vi "Spatial Dual Main (VISA).vi"(6 "Queue in":refnum<queue>, 7 "error in":errorcluster) -> (0 "error out":errorcluster)   [LabVIEW 2019]
uses:
  Globals and Definitions/System Message.ctl
  Globals and Definitions/Serial - Settings.ctl
  Globals and Definitions/Enum_FileNewInterval.ctl
  Globals and Definitions/RT Globals RD v1.0.vi
  <vilib>/Instr/_visa.llb/VISA Configure Serial Port (Instr).vi
  Globals and Definitions/Initialization Globals.vi
  <vilib>/Utility/file.llb/Write Delimited Spreadsheet (string).vi
  SpatialDual_Parsers.lvlib
panel:
  in  "Read Count":u32=1000
  in  "Termination Character":u8=10 format="%.0x"
  in  "VISA resource name":refnum<visa-resource-name>="COM1"
  in  "Serial Settings":T1={"baud rate"=9600, "data bits"=8, "parity"=enum."None", "stop bits"=10, "flow control"=0} {"flow control" items=["None"=0, "XON/XOFF"=1, "RTS/CTS"=2, "DTR/DSR"=4]; "stop bits" items=["1.0"=10, "1.5"=15, "2.0"=20]; "data bits" min=5 max=8 step=1; "baud rate" items=["75"=75, "110"=110, "134"=134, "150"=150, "300"=300, "600"=600, "1200"=1200, "1800"=1800, "2400"=2400, "4800"=4800, "7200"=7200, "9600"=9600, "14400"=14400, "19200"=19200, "28800"=28800, "38400"=38400, "56000"=56000, "57600"=57600, "115200"=115200, "128000"=128000, "230400"=230400]}
  out "Unix Timestamp":u64
  out "INS Filter Status Array":bool[](array[boolean])
  out "Packet 20 Decoded Data Cluster":T2
  in  "String Precision":i16=6
  out "size(s)":i32
  out "Packet Size":u8
  out "Packet ID":u8
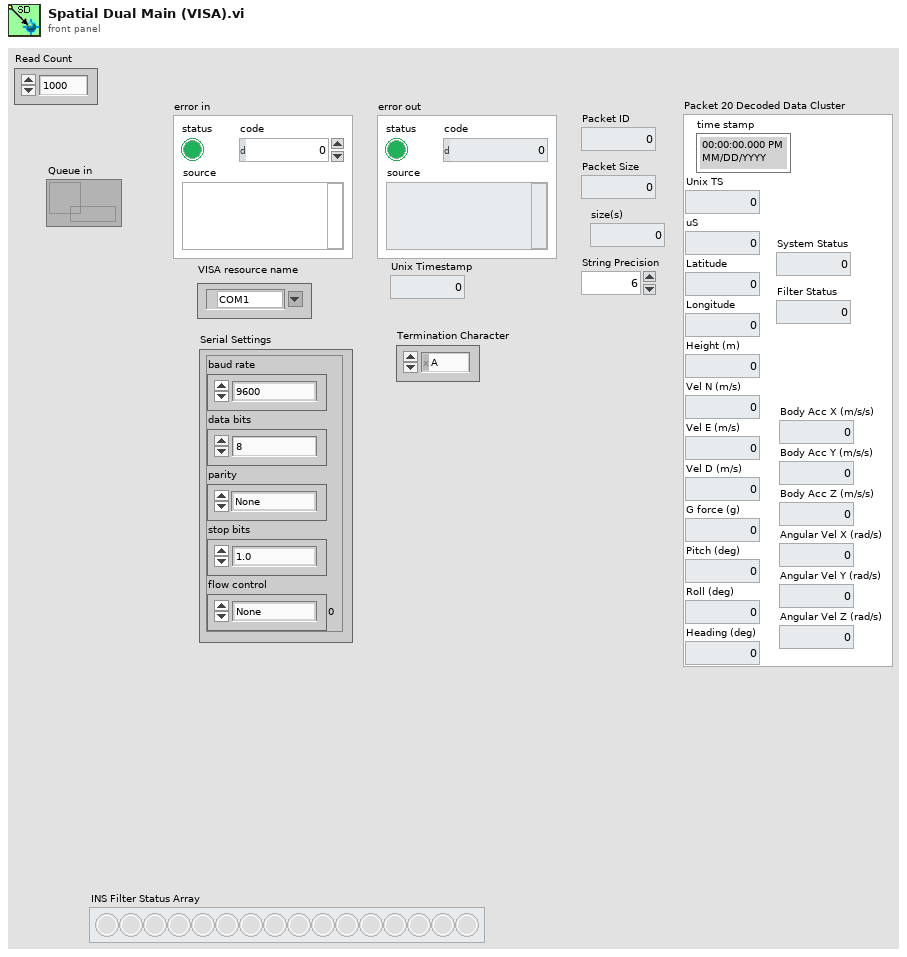
[diagram p1: front panel]
types:
  T1 = typedef "Serial - Settings.ctl" = cluster{"baud rate":u32, "data bits":u16, "parity":enum16{"None", "Odd", "Even", "Mark", "Space"}, "stop bits":u16, "flow control":u16}
  T2 = cluster{"time stamp":timestamp, "Unix TS":u32, "uS":u32, "Latitude":dbl, "Longitude":dbl, "Height (m)":dbl, "Vel N (m/s)":sgl, "Vel E (m/s)":sgl, "Vel D (m/s)":sgl, "G force (g)":sgl, "Pitch (deg)":sgl, "Roll (deg)":sgl, "Heading (deg)":sgl, "Body Acc X (m/s/s)":sgl, "Body Acc Y (m/s/s)":sgl, "Body Acc Z (m/s/s)":sgl, "Angular Vel X (rad/s)":sgl, "Angular Vel Y (rad/s)":sgl, "Angular Vel Z (rad/s)":sgl, "Filter Status":u16, "System Status":u16}
  T3 = enum16{"CRC Check", "Load Packet", "LRC Check", "Prescan Stream"}
  T4 = typedef "System Message.ctl" = cluster{"Message Tag":string, "Message Body":string, "Snooze Time (s)":dbl, "Snooze Alert?":bool, "Log Event?":bool, "Send Email":i32}
  T5 = typedef "Enum_FileNewInterval.ctl" = enum16{"10 Min", "Hourly", "Daily", "Weekly", "Monthly"}
  T6 = cluster{"All Data Types":string[], "All Units":string[], "All Names":string[], "Group Name":string}
  T7 = cluster{"Unix TS":u32, "uS":u32, "Latitude":dbl, "Longitude":dbl, "Height (m)":dbl, "Vel N (m/s)":sgl, "Vel E (m/s)":sgl, "Vel D (m/s)":sgl, "G force (g)":sgl, "Pitch (deg)":sgl, "Roll (deg)":sgl, "Heading (deg)":sgl, "Body Acc X (m/s/s)":sgl, "Body Acc Y (m/s/s)":sgl, "Body Acc Z (m/s/s)":sgl, "Angular Vel X (rad/s)":sgl, "Angular Vel Y (rad/s)":sgl, "Angular Vel Z (rad/s)":sgl, "Filter Status":u16, "System Status":u16}
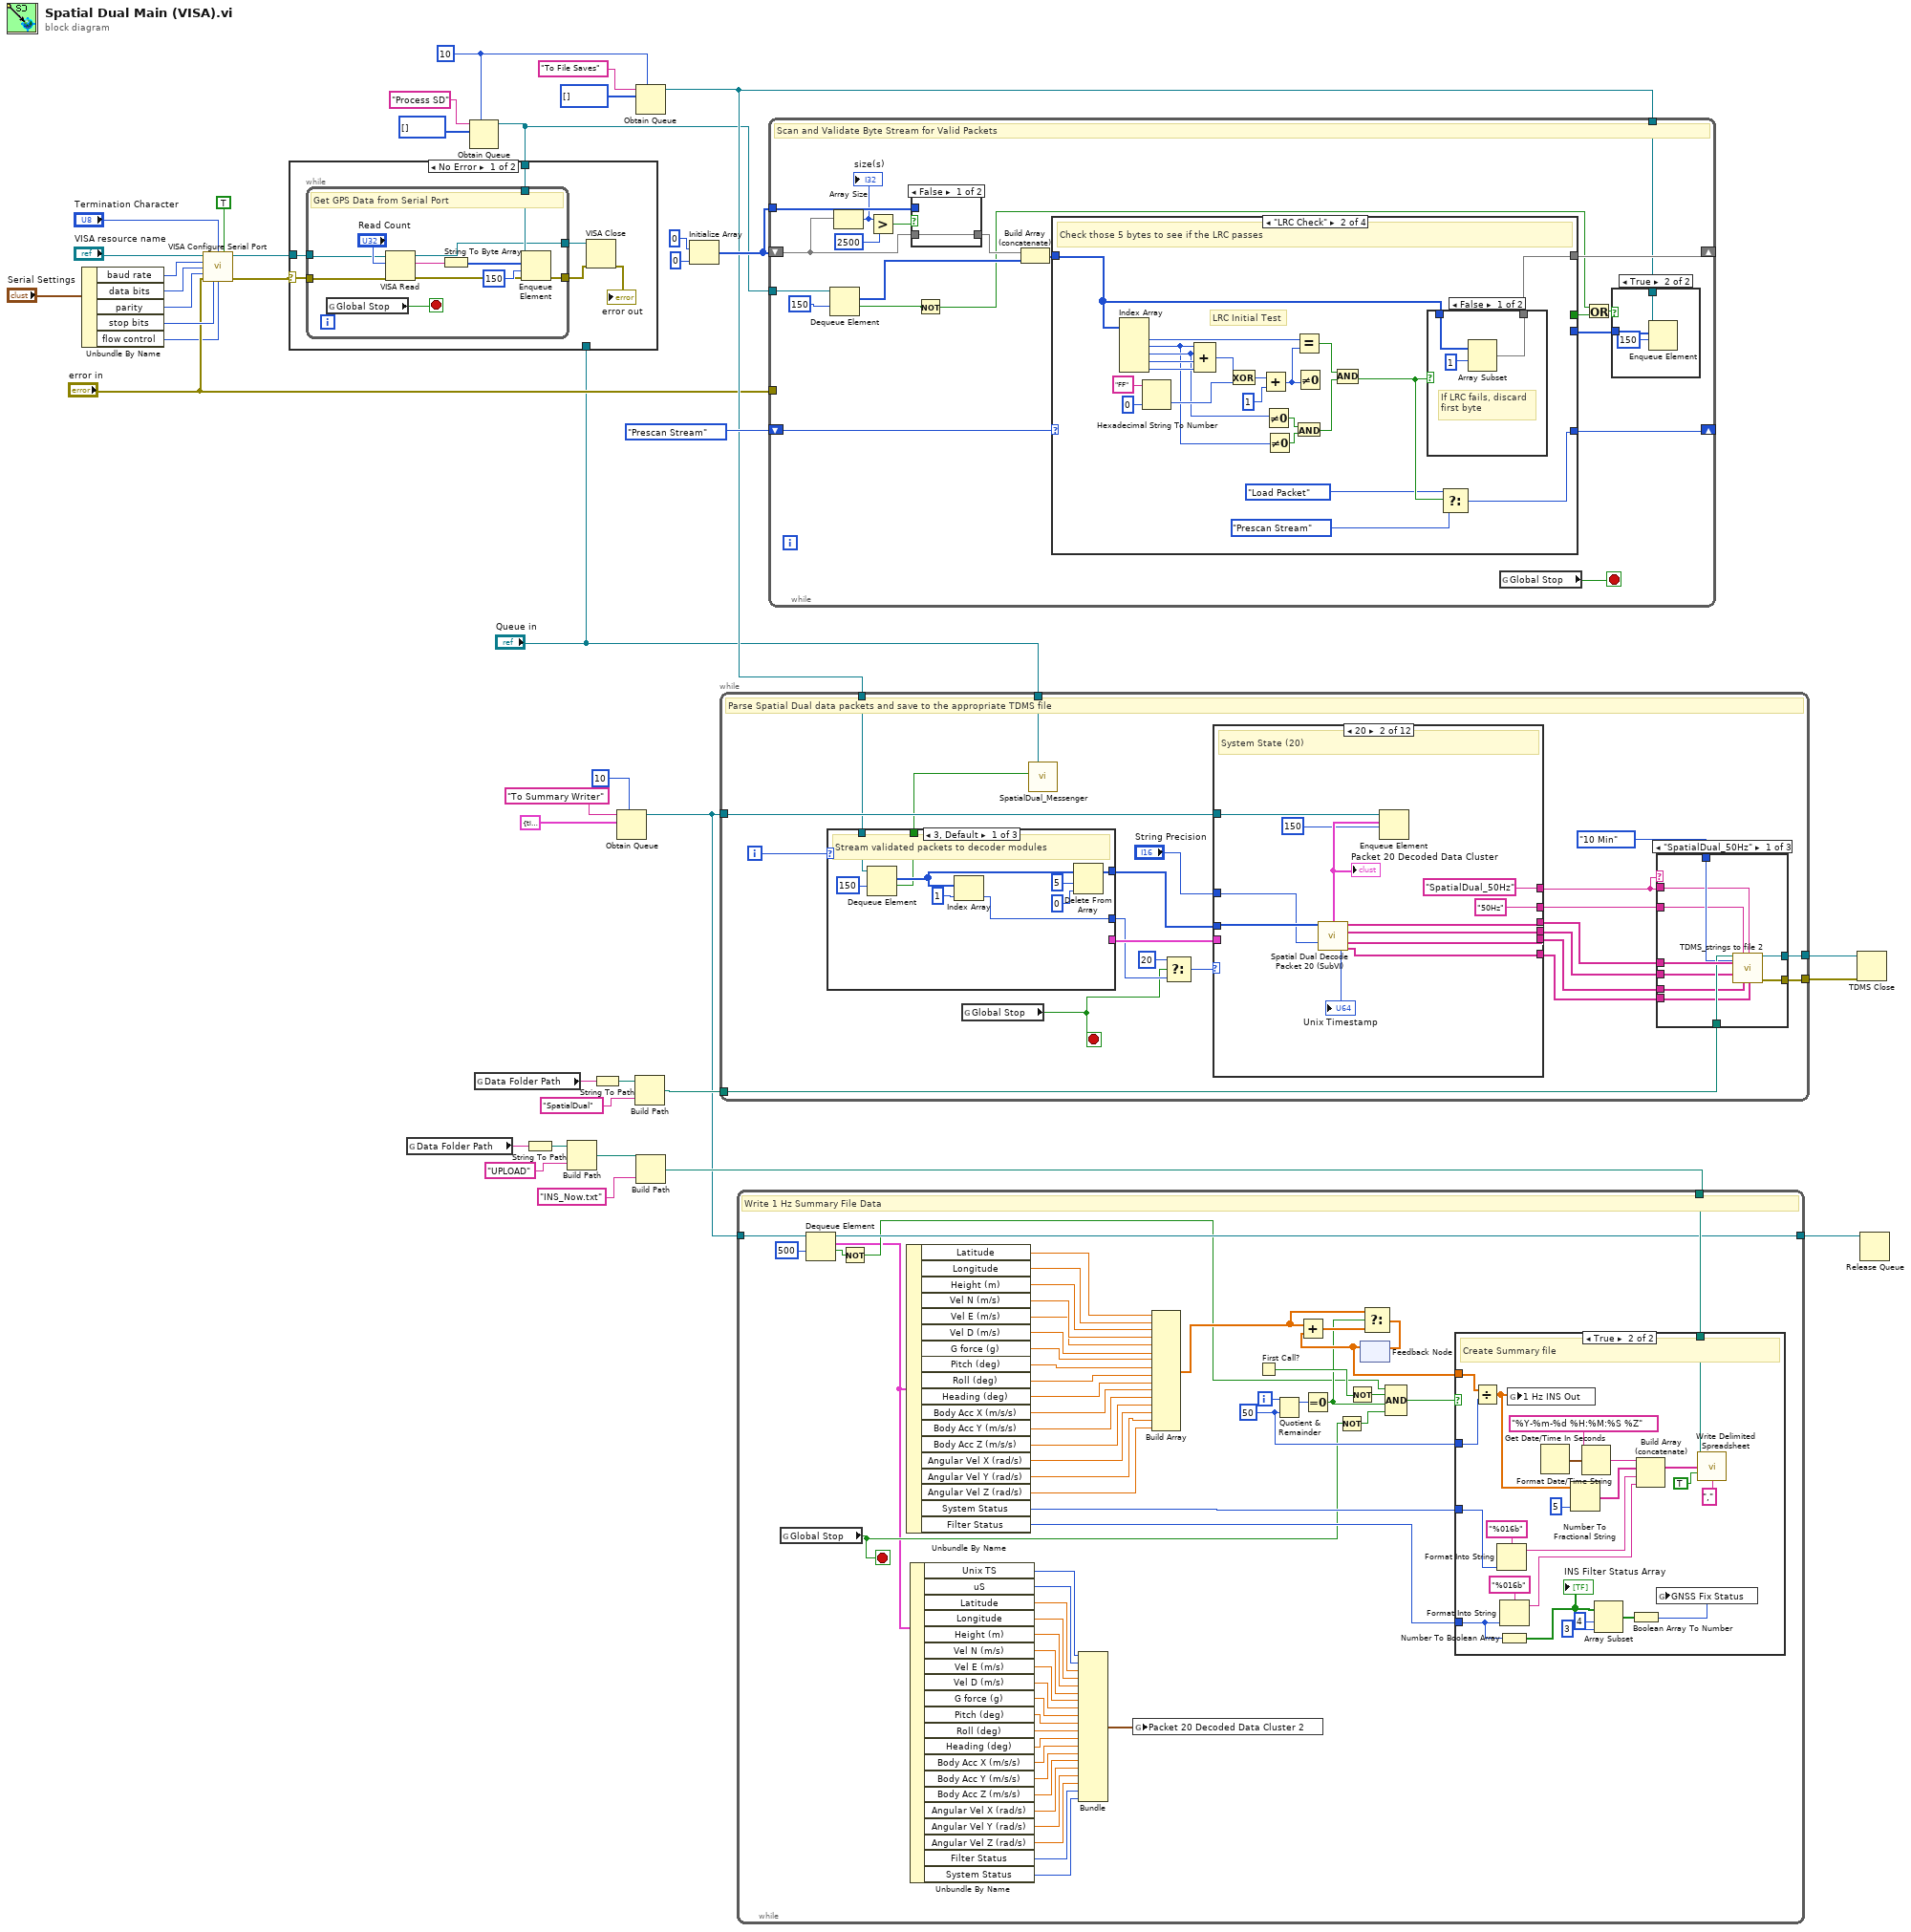
[diagram p0: block diagram]
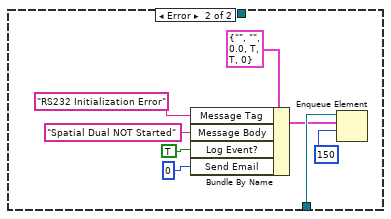
[diagram p2: hidden frame]
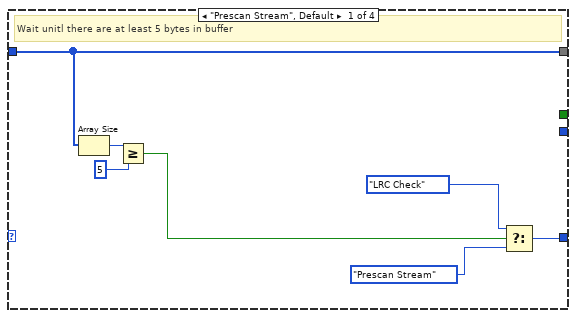
[diagram p6: hidden frame]
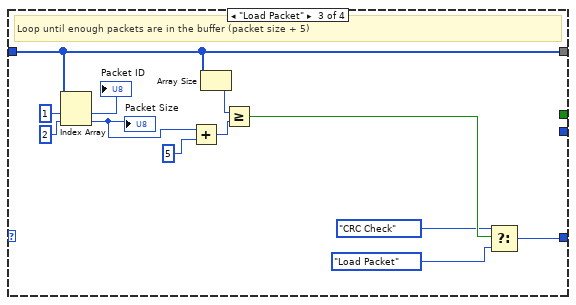
[diagram p8: hidden frame]
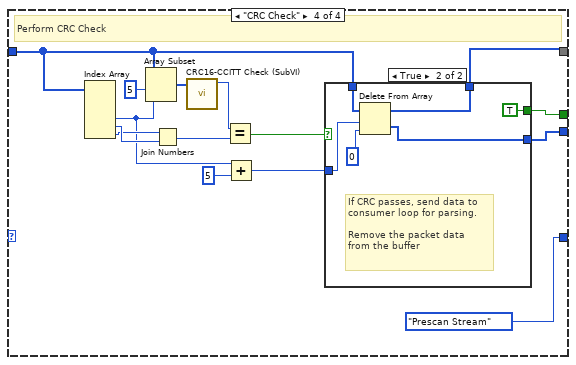
[diagram p9: hidden frame]
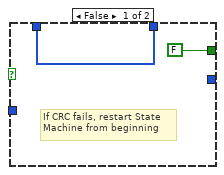
[diagram p10: hidden frame]
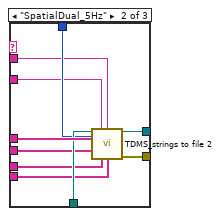
[diagram p11: hidden frame]
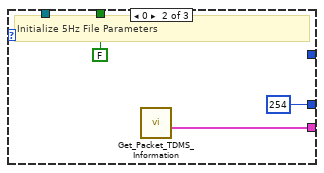
[diagram p13: hidden frame]
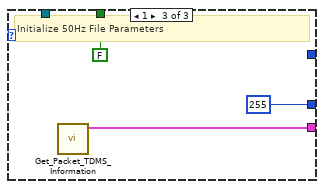
[diagram p14: hidden frame]
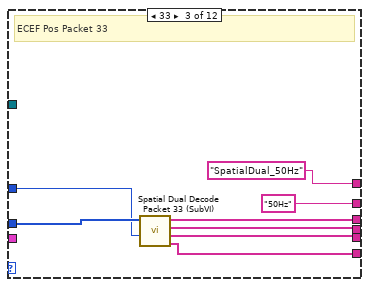
[diagram p16: hidden frame]
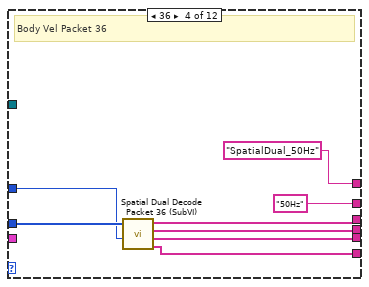
[diagram p17: hidden frame]
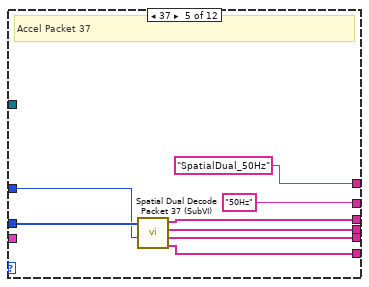
[diagram p18: hidden frame]
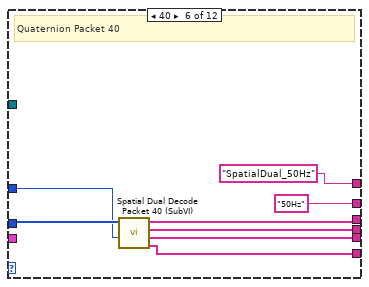
[diagram p19: hidden frame]
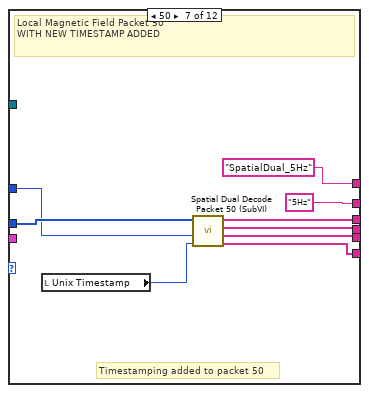
[diagram p20: hidden frame]
diagram:
  w15 = 10 ("max queue size (-1, unlimited)")
  n1 = Unbundle By Name("Serial Settings") -> ("baud rate"=w12:u32, "data bits"=w11:u16, "parity"=w10:enum16{"None", "Odd", "Even", "Mark", "Space"}, "stop bits"=w9:u16, "flow control"=w4:u16)
  n2 = call-poly "VISA Configure Serial Port"("VISA resource name"="VISA resource name", "termination char\n(0xA = '\\n' = LF)"="Termination Character", "Enable Termination\nChar (T)"=TRUE ("Enable Termination\nChar (T)"), "baud rate (9600)"=w12, "data bits (8)"=w11, "parity (0:none)"=w10, "error in (no error)"="error in", "stop bits (10: 1 bit)"=w9, "flow control (0:none)"=w4) -> ("VISA resource name out"=w3:refnum<visa-resource-name>, "error out"=w2:errorcluster)  [unwired: 1 in, 4 out]
  n3 = global read "Initialization Globals.vi" "Data Folder Path"() -> (w29:string)
  n4 = Obtain Queue(max queue size (-1, unlimited)=w15, name (unnamed)="Process SD", element data type=u8[] [] ("appended array")) -> (queue out=w16:refnum<queue>)  [unwired: 2 in, 2 out]
  n5 = case shown="No Error" w2 {
    selector: w2 -> [w42 _]
    tunnel: w16 -> [w47 _]
    tunnel: w3 -> [w46 _]
    tunnel: "Queue in" -> [_ w63]
    frame No Error {
      n6 = while {
        tunnel: w47 -> [w57]
        tunnel: w42 -> [w51]
        tunnel: w46 -> [w54]
        tunnel: [w49] -> w45
        tunnel: [w48] -> w44
        stop <- w58 stop-if-true
        # "Get GPS Data from Serial Port"
        n7 = global read "RT Globals RD v1.0.vi" "Global Stop"() -> (w58:bool)
        n8 = VISA Read(VISA resource name=w54, byte count="Read Count", error in (no error)=w51) -> (VISA resource name out=w49:refnum<visa-resource-name>, read buffer=w53:string, error out=w50:errorcluster)  [unwired: 1 out]
        n9 = String To Byte Array(string=w53) -> (unsigned byte array=w52:u8[])
        n10 = Enqueue Element(queue=w57, element=w52, timeout in ms (-1)=150, error in (no error)=w50) -> (error out=w48:errorcluster)  [unwired: 2 out]
      }
      n11 = VISA Close(VISA resource name=w45, error in (no error)=w44) -> (error out=→"error out":errorcluster)
    }
    frame Error {
      n12 = Bundle By Name(cluster=T4 {"Message Tag"="", "Message Body"="", "Snooze Time (s)"=0.0, "Snooze Alert?"=TRUE, "Log Event?"=TRUE, "Send Email"=0}, "Message Tag"="RS232 Initialization Error", "Message Body"="Spatial Dual NOT Started", "Log Event?"=TRUE, "Send Email"=0) -> (w62:T4)
      n13 = Enqueue Element(queue=w63, element=w62, timeout in ms (-1)=150) -> ()  [unwired: 1 in, 3 out]
    }
  }
  n14 = global read "Initialization Globals.vi" "Data Folder Path"() -> (w33:string)
  n15 = String To Path(string=w29) -> (path=w30:path)
  n16 = Build Path(base path=w30, name or relative path="UPLOAD") -> (appended path=w27:path)
  n17 = String To Path(string=w33) -> (path=w34:path)
  n18 = Obtain Queue(max queue size (-1, unlimited)=10, name (unnamed)="To Summary Writer", element data type=T2 {"time stamp"=timestamp(0 s since 1904-01-01), "Unix TS"=0, "uS"=0, "Latitude"=0.0, "Longitude"=0.0, "Height (m)"=0.0, "Vel N (m/s)"=0.0, "Vel E (m/s)"=0.0, "Vel D (m/s)"=0.0, "G force (g)"=0.0, "Pitch (deg)"=0.0, "Roll (deg)"=0.0, "Heading (deg)"=0.0, "Body Acc X (m/s/s)"=0.0, "Body Acc Y (m/s/s)"=0.0, "Body Acc Z (m/s/s)"=0.0, "Angular Vel X (rad/s)"=0.0, "Angular Vel Y (rad/s)"=0.0, "Angular Vel Z (rad/s)"=0.0, "Filter Status"=0, "System Status"=0} ("Packet 20 Decoded Data Cluster 2")) -> (queue out=w24:refnum<queue>)  [unwired: 2 in, 2 out]
  n19 = Build Path(base path=w34, name or relative path="SpatialDual") -> (appended path=w32:path)
  n20 = Obtain Queue(max queue size (-1, unlimited)=w15, name (unnamed)="To File Saves", element data type=u8[] []) -> (queue out=w19:refnum<queue>)  [unwired: 2 in, 2 out]
  n21 = Build Path(base path=w27, name or relative path="INS_Now.txt") -> (appended path=w26:path)
  n22 = Initialize Array(u8 0, 0 ("dimension size")) -> (w39:u8[])
  n23 = while {
    tunnel: w32 -> [w84]
    tunnel: [w87] -> w37
    tunnel: [w86] -> w36
    tunnel: w24 -> [w71]
    tunnel: "Queue in" -> [w69]
    tunnel: w19 -> [w68]
    i -> [w76]
    stop <- w67 stop-if-true
    # "Parse Spatial Dual data packets and save to the appropriate TDMS file"
    n24 = case shown="3, Default" w76 {
      tunnel: [w114 _ _] -> w88
      tunnel: [w113 u8 254 u8 255] -> w72
      tunnel: [_ w120 w122] -> w77
      tunnel: [w110 FALSE ("timed out?") FALSE ("timed out?")] -> w70
      tunnel: w68 -> [w112 _ _]
      frame 3, Default {
        # "Stream validated packets to decoder modules"
        n25 = Dequeue Element(queue=w112, timeout in ms (-1)=150) -> (element=w111:u8[], timed out?=w110:bool)  [unwired: 1 in, 2 out]
        n26 = Index Array(array=w111, index=1) -> (element=w113:u8)
        n27 = Delete From Array(array=w111, length=5, index=0) -> (array with subset deleted=w114:u8[])  [unwired: 1 out]
      }
      frame 0 {
        # "Initialize 5Hz File Parameters"
        n28 = call "Get_Packet_TDMS_Information.vi"() -> ("TDMS Info 5Hz"=w120:T6)  [unwired: 10 in, 1 out]
      }
      frame 1 {
        # "Initialize 50Hz File Parameters"
        n29 = call "Get_Packet_TDMS_Information.vi"() -> ("TDMS Info 50Hz"=w122:T6)  [unwired: 10 in, 1 out]
      }
    }
    n30 = global read "RT Globals RD v1.0.vi" "Global Stop"() -> (w67:bool)
    n31 = call "SpatialDual_Messenger.vi"("Queue in"=w69, "Time Out"=w70) -> ()  [unwired: 10 in]
    n32 = Select(t=20, s=w67, f=w72) -> (s? t:f=w74:i32)
    n33 = case shown="20" w74 {
      tunnel: w88 -> [_ w135 w143 w151 w159 w167 w175 w183 w191 w200 _ _]
      tunnel: [_ w134 w141 w149 w158 w165 w173 w181 w189 w198 w204 w212] -> w85
      tunnel: [_ w133 w140 w148 w157 w164 w172 w180 w188 w197 _ _] -> w83
      tunnel: [_ w132 w139 w147 w156 w163 w171 w179 w187 w196 w203 w211] -> w82
      tunnel: [_ w131 w138 w146 w155 w162 w170 w178 w186 w195 w202 w210] -> w81
      tunnel: [_ "50Hz" ("FileName") "50Hz" ("FileName") "50Hz" ("FileName") "50Hz" ("FileName") "50Hz" ("FileName") "5Hz" ("FileName") "5Hz" ("FileName") "50Hz" ("FileName") "5Hz" ("FileName") w205 w209] -> w79
      tunnel: "String Precision" -> [_ w129 w142 w150 w153 w166 w174 w182 w190 w199 _ _]
      tunnel: w77 -> [_ _ _ _ _ _ _ _ _ _ w206 w207]
      tunnel: [_ "SpatialDual_50Hz" ("FileName") "SpatialDual_50Hz" ("FileName") "SpatialDual_50Hz" ("FileName") "SpatialDual_50Hz" ("FileName") "SpatialDual_50Hz" ("FileName") "SpatialDual_5Hz" ("FileName") "SpatialDual_5Hz" ("FileName") "SpatialDual_50Hz" ("FileName") "SpatialDual_5Hz" ("FileName") "SpatialDual_5Hz" ("FileName") "SpatialDual_50Hz" ("FileName")] -> w75
      tunnel: w71 -> [_ w127 _ _ _ _ _ _ _ _ _ _]
      frame 0, Default {
      }
      frame 20 {
        # "System State (20)"
        n34 = call "Spatial Dual Decode Packet 20 (SubVI).vi"("Packet 20 Bytes In"=w135, "String Precision"=w129) -> ("Packet 20 Decoded Data Cluster"=w126:T2, "Channel Names"=w134:string[], "Data"=w133:string[], "Channel Units"=w132:string[], "Unix Timestamp"=→"Unix Timestamp":u64, "Data Types"=w131:string[])  [unwired: 8 in]
        "Packet 20 Decoded Data Cluster" <- w126
        n35 = Enqueue Element(queue=w127, element=w126, timeout in ms (-1)=150) -> ()  [unwired: 1 in, 3 out]
      }
      frame 33 {
        # "ECEF Pos Packet 33"
        n36 = call "Spatial Dual Decode Packet 33 (SubVI).vi"("SGL Precision"=w142, "Packet 33 Bytes In"=w143) -> ("Channel Data Type"=w138:string[], "Channel Units"=w139:string[], "Data"=w140:string[], "Channel Names"=w141:string[])  [unwired: 4 in, 1 out]
      }
      frame 36 {
        # "Body Vel Packet 36"
        n37 = call "Spatial Dual Decode Packet 36 (SubVI).vi"("SGL Precision"=w150, "Packet 36 Bytes In"=w151) -> ("Channel Data Type"=w146:string[], "Channel Units"=w147:string[], "Data"=w148:string[], "Channel Names"=w149:string[])  [unwired: 4 in, 1 out]
      }
      frame 37 {
        # "Accel Packet 37"
        n38 = call "Spatial Dual Decode Packet 37 (SubVI).vi"("SGL Precision"=w153, "Packet 37 Bytes In"=w159) -> ("Channel Data Type"=w155:string[], "Channel Units"=w156:string[], "Data"=w157:string[], "Channel Names"=w158:string[])  [unwired: 4 in, 1 out]
      }
      frame 40 {
        # "Quaternion Packet 40"
        n39 = call "Spatial Dual Decode Packet 40 (SubVI).vi"("SGL Precision"=w166, "Packet 40 Bytes In"=w167) -> ("Channel Data Type"=w162:string[], "Channel Units"=w163:string[], "Data"=w164:string[], "Channel Names"=w165:string[])  [unwired: 4 in, 1 out]
      }
      frame 50 {
        # "Timestamping added to packet 50"
        # "Local Magnetic Field Packet 50\nWITH NEW TIMESTAMP ADDED"
        n40 = local read "Unix Timestamp"() -> (w168:u64)
        n41 = call "Spatial Dual Decode Packet 50 (SubVI).vi"("Unix Timestamp"=w168, "SGL Precision"=w174, "Packet 50 Bytes In"=w175) -> ("Channel Data Type"=w170:string[], "Channel Units"=w171:string[], "Data"=w172:string[], "Channel Names"=w173:string[])  [unwired: 3 in, 1 out]
      }
      frame 54 {
        # "Geoid Height Packet 54"
        n42 = call "Spatial Dual Decode Packet 54 (SubVI).vi"("SGL Precision"=w182, "Packet 54 Bytes In"=w183) -> ("Channel Data Type"=w178:string[], "Channel Units"=w179:string[], "Data"=w180:string[], "Channel Names"=w181:string[])  [unwired: 4 in, 1 out]
      }
      frame 58 {
        # "Heave Packet 58"
        n43 = call "Spatial Dual Decode Packet 58 (SubVI).vi"("SGL Precision"=w190, "Packet 58 Bytes In"=w191) -> ("Channel Data Type"=w186:string[], "Channel Units"=w187:string[], "Data"=w188:string[], "Channel Names"=w189:string[])  [unwired: 4 in, 1 out]
      }
      frame 85 {
        # "Sensor Temps Packets 85"
        n44 = call "Spatial Dual Decode Packet 85 (SubVI).vi"("SGL Precision"=w199, "Packet 85 Bytes In"=w200) -> ("Channel Data Type"=w195:string[], "Channel Units"=w196:string[], "Data"=w197:string[], "Channel Names"=w198:string[])  [unwired: 4 in, 1 out]
      }
      frame 254 {
        # "Start 5Hz File"
        n45 = Unbundle By Name(w206) -> ("Group Name"=w205:string, "All Names"=w204:string[], "All Units"=w203:string[], "All Data Types"=w202:string[])
      }
      frame 255 {
        # "Start 50Hz file"
        n46 = Unbundle By Name(w207) -> ("Group Name"=w209:string, "All Names"=w212:string[], "All Units"=w211:string[], "All Data Types"=w210:string[])
      }
    }
    n47 = case shown="\"SpatialDual_50Hz\"" w75 {
      tunnel: [w98 w108 _] -> w87
      tunnel: [w97 w107 _] -> w86
      tunnel: w85 -> [w96 w106 _]
      tunnel: w84 -> [w95 w105 _]
      tunnel: w83 -> [w94 w104 _]
      tunnel: w82 -> [w93 w103 _]
      tunnel: w81 -> [w92 w102 _]
      tunnel: Enum_FileNewInterval."10 Min" ("Interval") -> [w91 w101 _]
      tunnel: w79 -> [w90 w100 _]
      tunnel: w75 -> [w89 w99 _]
      frame "SpatialDual_50Hz" {
        n48 = call "TDMS_strings to file 2.vi"("Base path"=w95, "Group Name"=w90, "FileName"=w89, "Interval"=w91, "Channel Names"=w96, "Data"=w94, "Channel Units"=w93, "property Metadata"=w92) -> ("file out"=w98:refnum<k34>, "error out"=w97:errorcluster)  [unwired: 6 in]
      }
      frame "SpatialDual_5Hz" {
        n49 = call "TDMS_strings to file 2.vi"("Base path"=w105, "Group Name"=w100, "FileName"=w99, "Interval"=w101, "Channel Names"=w106, "Data"=w104, "Channel Units"=w103, "property Metadata"=w102) -> ("file out"=w108:refnum<k34>, "error out"=w107:errorcluster)  [unwired: 6 in]
      }
      frame Default {
      }
    }
  }
  n50 = while {
    tunnel: w26 -> [w248]
    tunnel: w24 -> [w240]
    tunnel: [w237] -> w23
    i -> [w252]
    stop <- w238 stop-if-true
    w250 = 50
    # "Write 1 Hz Summary File Data"
    n51 = global read "RT Globals RD v1.0.vi" "Global Stop"() -> (w238:bool)
    n52 = Dequeue Element(queue=w240, timeout in ms (-1)=500) -> (queue out=w237:refnum<queue>, element=w234:T2, timed out?=w236:bool)  [unwired: 1 in, 1 out]
    n53 = Not(x=w236) -> (.not. x?=w235:bool)
    n54 = Unbundle By Name(w234) -> ("Latitude"=w249:dbl, "Longitude"=w271:dbl, "Height (m)"=w270:dbl, "Vel N (m/s)"=w269:sgl, "Vel E (m/s)"=w268:sgl, "Vel D (m/s)"=w267:sgl, "G force (g)"=w266:sgl, "Pitch (deg)"=w265:sgl, "Roll (deg)"=w264:sgl, "Heading (deg)"=w263:sgl, "Body Acc X (m/s/s)"=w262:sgl, "Body Acc Y (m/s/s)"=w261:sgl, "Body Acc Z (m/s/s)"=w260:sgl, "Angular Vel X (rad/s)"=w259:sgl, "Angular Vel Y (rad/s)"=w258:sgl, "Angular Vel Z (rad/s)"=w257:sgl, "System Status"=w242:u16, "Filter Status"=w243:u16)
    n55 = Unbundle By Name(w234) -> ("Unix TS"=w233:u32, "uS"=w232:u32, "Latitude"=w231:dbl, "Longitude"=w230:dbl, "Height (m)"=w229:dbl, "Vel N (m/s)"=w228:sgl, "Vel E (m/s)"=w227:sgl, "Vel D (m/s)"=w226:sgl, "G force (g)"=w225:sgl, "Pitch (deg)"=w224:sgl, "Roll (deg)"=w223:sgl, "Heading (deg)"=w222:sgl, "Body Acc X (m/s/s)"=w221:sgl, "Body Acc Y (m/s/s)"=w220:sgl, "Body Acc Z (m/s/s)"=w219:sgl, "Angular Vel X (rad/s)"=w218:sgl, "Angular Vel Y (rad/s)"=w217:sgl, "Angular Vel Z (rad/s)"=w216:sgl, "Filter Status"=w215:u16, "System Status"=w214:u16)
    n56 = Bundle("Unix TS"=w233, "uS"=w232, "Latitude"=w231, "Longitude"=w230, "Height (m)"=w229, "Vel N (m/s)"=w228, "Vel E (m/s)"=w227, "Vel D (m/s)"=w226, "G force (g)"=w225, "Pitch (deg)"=w224, "Roll (deg)"=w223, "Heading (deg)"=w222, "Body Acc X (m/s/s)"=w221, "Body Acc Y (m/s/s)"=w220, "Body Acc Z (m/s/s)"=w219, "Angular Vel X (rad/s)"=w218, "Angular Vel Y (rad/s)"=w217, "Angular Vel Z (rad/s)"=w216, "Filter Status"=w215, "System Status"=w214) -> (w213:T7)  [unwired: 1 in]
    n57 = global write "RT Globals RD v1.0.vi" "Packet 20 Decoded Data Cluster 2"(w213) -> ()
    n58 = Build Array(w249, w271, w270, w269, w268, w267, w266, w265, w264, w263, w262, w261, w260, w259, w258, w257) -> (w254:dbl[])
    n59 = First Call?() -> (First Call?: T/F=w247:bool)
    n60 = Quotient & Remainder(x=w252, y=w250) -> (x-y*floor(x/y)=w253:i32)  [unwired: 1 out]
    n61 = Equal To 0?(x=w253) -> (x = 0?=w245:bool)
    n62 = Not(x=w238) -> (.not. x?=w241:bool)
    n63 = Not(x=w247) -> (.not. x?=w246:bool)
    n64 = feedback #1() -> (w251:dbl[])  [unwired: 1 in]
    n65 = Add(x=w254, y=w251) -> (x+y=w256:dbl[])
    n66 = Select(t=w254, s=w245, f=w256) -> (s? t:f=w255:dbl[])
    n67 = feedback-in #1(w255) -> ()
    n68 = Compound Arithmetic op=AND(w235, w246, w245, w241) -> (w244:bool)
    n69 = case shown="True" w244 {
      tunnel: w251 -> [_ w294]
      tunnel: w250 -> [_ w293]
      tunnel: w248 -> [_ w283]
      tunnel: w243 -> [_ w274]
      tunnel: w242 -> [_ w280]
      frame False {
      }
      frame True {
        # "Create Summary file"
        n70 = Divide(x=w294, y=w293) -> (x/y=w288:dbl[])
        n71 = Format Into String(format string="%016b", w280) -> (resulting string=w279:string)  [unwired: 2 in, 1 out]
        n72 = Format Into String(format string="%016b", w274) -> (resulting string=w278:string)  [unwired: 2 in, 1 out]
        n73 = Number To Boolean Array(number=w274) -> (Boolean array=w273:bool[])
        "INS Filter Status Array" <- w273
        n74 = global write "RT Globals RD v1.0.vi" "1 Hz INS Out"(w288) -> ()
        n75 = Get Date/Time In Seconds() -> (seconds since 1Jan1904=w291:timestamp)
        n76 = Number To Fractional String(number=w288, precision (6)=i16 5) -> (F-format string=w287:string[])  [unwired: 2 in]
        n77 = Format Date/Time String(time format string (%c)="%Y-%m-%d %H:%M:%S %Z", seconds (now)=w291) -> (date/time string=w290:string)  [unwired: 1 in]
        n78 = Array Subset(array=w273, index=4, length=3) -> (w277:bool[])
        n79 = Boolean Array To Number(Boolean array=w277) -> (number=w272:u32)
        n80 = Build Array (concatenate)(w290, w287, w279, w278) -> (w284:string[])
        n81 = global write "RT Globals RD v1.0.vi" "GNSS Fix Status"(w272) -> ()
        n82 = call-poly <vilib>:"Write Delimited Spreadsheet.vi"("file path (dialog if empty)"=w283, "1D data"=w284, "append to file? (new file:F)"=TRUE, "delimiter (\\t)"="," ("delimiter (\\t)")) -> ()  [unwired: 10 in, 2 out]
      }
    }
  }
  n83 = while {
    shift-right: [w311] -> _
    shift-left: w39 -> [w308]
    shift-right: [w313] -> _
    shift-left: T3."Prescan Stream" -> [w314]
    tunnel: w39 -> [w309]
    tunnel: "error in" -> [_]
    tunnel: w19 -> [w301]
    tunnel: w16 -> [w299]
    stop <- w297 stop-if-true
    # "Scan and Validate Byte Stream for Valid Packets"
    n84 = Dequeue Element(queue=w299, timeout in ms (-1)=150) -> (element=w298:u8[], timed out?=w295:bool)  [unwired: 1 in, 2 out]
    n85 = Array Size(array=w308) -> (size(s)=w304:i32)
    "size(s)" <- w304
    n86 = Greater?(x=w304, y=2500) -> (0:w303:bool)
    n87 = case shown="False" w303 {
      tunnel: w309 -> [_ w319]
      tunnel: w308 -> [w318 _]
      tunnel: [w318 w319] -> w307
      frame False {
      }
      frame True {
      }
    }
    n88 = Not(x=w295) -> (.not. x?=w296:bool)
    n89 = Build Array (concatenate)(w307, w298) -> (w312:u8[])
    n90 = case shown="\"LRC Check\"" w314 {
      tunnel: [w324 w327 w355 T3."Prescan Stream"] -> w313
      tunnel: w312 -> [w322 w331 w362 w374]
      tunnel: [w322 w338 w362 w373] -> w311
      tunnel: [_ _ _ w369] -> w306
      tunnel: [_ _ _ w368] -> w305
      frame "Prescan Stream", Default {
        # "Wait unitl there are at least 5 bytes in buffer"
        n91 = Array Size(array=w322) -> (size(s)=w326:i32)
        n92 = Greater Or Equal?(x=w326, y=5) -> (x >= y?=w323:bool)
        n93 = Select(t=T3."LRC Check", s=w323, f=T3."Prescan Stream") -> (s? t:f=w324:T3)
      }
      frame "LRC Check" {
        # "LRC Initial Test"
        # "Check those 5 bytes to see if the LRC passes"
        n94 = Index Array(array=w331) -> (element #1=w347:u8, element #2=w336:u8, element #3=w337:u8, element #4=w342:u8, element #5=w343:u8)  [unwired: 5 in]
        n95 = Hexadecimal String To Number(string="FF", default (0uL)=u8 0 ("default (0 U32)")) -> (number=w346:u8)  [unwired: 1 in, 1 out]
        n96 = Compound Arithmetic op=ADD(w336, w337, w342, w343) -> (w345:u8)
        n97 = Exclusive Or(1:w346, 2:w345) -> (0:w344:u8)
        n98 = Add(x=w344, y=u8 1 ("value")) -> (x+y=w348:u8)
        n99 = Not Equal To 0?(x=w337) -> (x != 0?=w334:bool)
        n100 = Not Equal To 0?(x=w336) -> (x != 0?=w335:bool)
        n101 = Equal?(x=w347, y=w348) -> (x = y?=w333:bool)
        n102 = And(x=w334, y=w335) -> (x .and. y?=w332:bool)
        n103 = Not Equal To 0?(x=w348) -> ()  [unwired: 1 out]
        n104 = Compound Arithmetic op=AND(w333, w332) -> (w330:bool)
        n105 = case shown="False" w330 {
          tunnel: w331 -> [w351 w352]
          tunnel: [w350 w352] -> w338
          frame False {
            # "If LRC fails, discard\nfirst byte"
            n106 = Array Subset(array=w351, index=1) -> (w350:u8[])  [unwired: 1 in]
          }
          frame True {
            # "If LRC passes, \npreserve message\nfor Load Packet\nCase"
          }
        }
        n107 = Select(t=T3."Load Packet", s=w330, f=T3."Prescan Stream") -> (s? t:f=w327:T3)
      }
      frame "Load Packet" {
        # "Loop until enough packets are in the buffer (packet size + 5)"
        n108 = Index Array(array=w362, index #1=1 ("index"), index #2=2 ("index")) -> (element #1=→"Packet ID":u8, element #2=w359:u8)
        "Packet Size" <- w359
        n109 = Add(x=w359, y=u8 5) -> (x+y=w358:u8)
        n110 = Array Size(array=w362) -> (size(s)=w361:i32)
        n111 = Greater Or Equal?(x=w361, y=w358) -> (x >= y?=w360:bool)
        n112 = Select(t=T3."CRC Check", s=w360, f=T3."Load Packet") -> (s? t:f=w355:T3)
      }
      frame "CRC Check" {
        # "Perform CRC Check"
        n113 = Index Array(array=w374) -> (element #3=w372:u8, element #4=w377:u8, element #5=w376:u8)  [unwired: 5 in, 2 out]
        n114 = Array Subset(array=w374, index=5, length=w372) -> (w378:u8[])
        n115 = Join Numbers(hi=w376, lo=w377) -> ((hi.lo)=w366:u16)
        n116 = call "CRC16-CCITT Check (SubVI).vi"("Data In (u8)"=w378) -> ("CRC Calc"=w375:u16)  [unwired: 10 in]
        n117 = Equal?(x=w375, y=w366) -> (x = y?=w367:bool)
        n118 = Add(x=w372, y=u8 5) -> (x+y=w370:u8)
        n119 = case shown="True" w367 {
          tunnel: w374 -> [w380 w385]
          tunnel: [w380 w382] -> w373
          tunnel: w370 -> [_ w387]
          tunnel: [_ w384] -> w369
          tunnel: [FALSE TRUE] -> w368
          frame False {
            # "If CRC fails, restart State\nMachine from beginning"
          }
          frame True {
            # "If CRC passes, send data to \nconsumer loop for parsing.\n\nRemove the packet data \nfrom the buffer"
            n120 = Delete From Array(array=w385, length=w387, index=0) -> (deleted portion=w384:u8[], array with subset deleted=w382:u8[])
          }
        }
      }
    }
    n121 = global read "RT Globals RD v1.0.vi" "Global Stop"() -> (w297:bool)
    n122 = Or(x=w296, y=w305) -> (x .or. y?=w302:bool)
    n123 = case shown="True" w302 {
      tunnel: w306 -> [_ w316]
      tunnel: w301 -> [_ w317]
      frame False {
      }
      frame True {
        n124 = Enqueue Element(queue=w317, element=w316, timeout in ms (-1)=150) -> ()  [unwired: 1 in, 3 out]
      }
    }
  }
  n125 = TDMS Close(8:w36, 11:w37) -> ()  [unwired: 2 out]
  n126 = Release Queue(queue=w23) -> ()  [unwired: 2 in, 3 out]
